vi "Proto Parser.vi"(8 "error in (no error)":errorcluster, 10 "Import Paths":path[](array[path]), 11 ".proto file path":path) -> (0 "error out":errorcluster, 1 "gRPC Method Parameters":T5[](array[typedef]), 2 "gRPC Enum Parameters":T1[](array[typedef]), 3 "gRPC Message Parameters":T2[](array[typedef]), 4 "Serialised Proto":string)   [LabVIEW 2019, in "gRPC Template Creation Utility.lvlib"]
uses:
  gRPC Template Creation Utility.lvlib
  TypeDefs/RPC Method Parameters.ctl
  TypeDefs/Message Metadata (Scripting).ctl
  TypeDefs/Message Element Metadata (Scripting).ctl
  TypeDefs/Message Element Type.ctl
  TypeDefs/Enum Metadata (Scripting).ctl
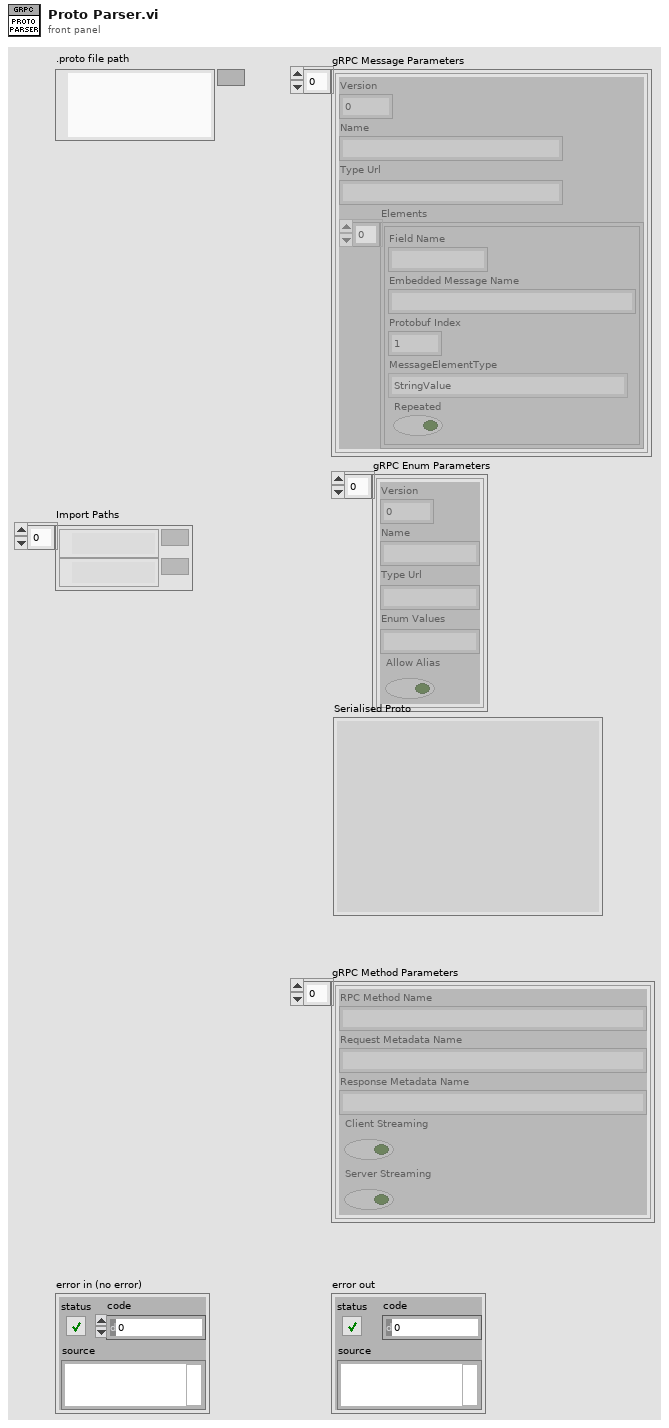
[diagram p1: front panel]
types:
  T1 = typedef "gRPC Template Creation Utility.lvlib/Enum Metadata (Scripting).ctl" = cluster{"Version":i32, "Name":string, "Type Url":string, "Enum Values":string, "Allow Alias":bool}
  T2 = typedef "gRPC Template Creation Utility.lvlib/Message Metadata (Scripting).ctl" = cluster{"Version":i32, "Name":string, "Type Url":string, "Elements":T3[]}
  T3 = typedef "gRPC Template Creation Utility.lvlib/Message Element Metadata (Scripting).ctl" = cluster{"Field Name":string, "Embedded Message Name":string, "Protobuf Index":i32, "MessageElementType":T4, "Repeated":bool}
  T4 = typedef "gRPC Template Creation Utility.lvlib/Message Element Type.ctl" = enum32{"Int32Value", "FloatValue", "DoubleValue", "BoolValue", "StringValue", "MessageValue", "Int64Value", "UInt32Value", "UInt64Value", "EnumValue", "Bytes", "Fixed64", "Fixed32", "SFixed64", "SFixed32", "SInt64", "SInt32"}
  T5 = typedef "gRPC Template Creation Utility.lvlib/RPC Method Parameters.ctl" = cluster{"RPC Method Name":string, "Request Metadata Name":string, "Response Metadata Name":string, "Client Streaming":bool, "Server Streaming":bool}
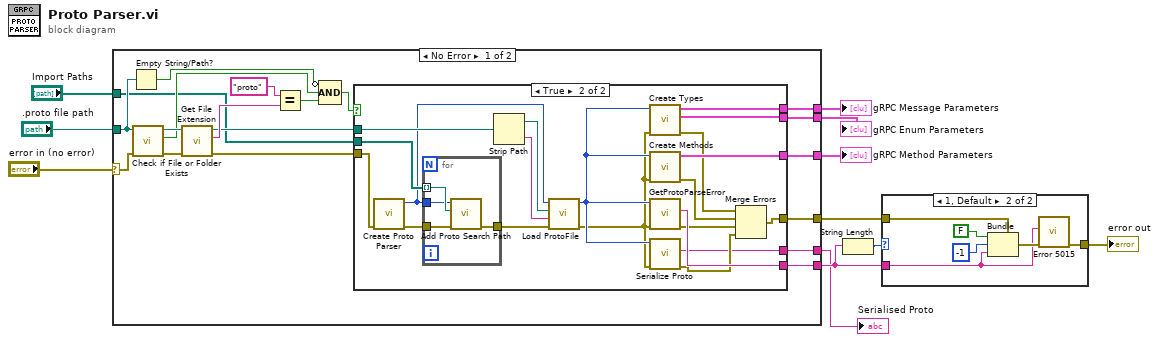
[diagram p0: block diagram]
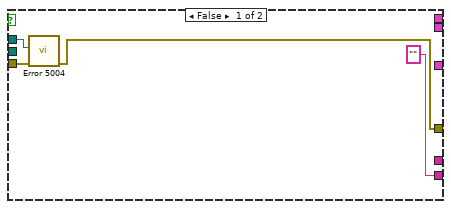
[diagram p3: hidden frame]
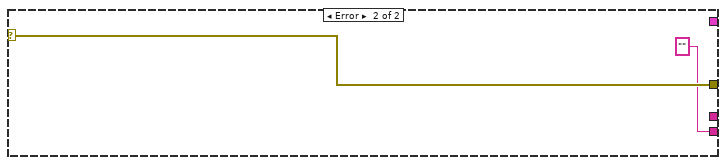
[diagram p4: hidden frame]
diagram:
  n1 = case shown="No Error" "error in (no error)" {
    selector: "error in (no error)" -> [w27 w60]
    tunnel: ".proto file path" -> [w28 _]
    tunnel: [w30 _] -> w11
    tunnel: [w29 w60] -> w5
    tunnel: [w16 _] -> w8
    tunnel: "Import Paths" -> [w15 _]
    tunnel: [w14 "" ("Error Message")] -> w3
    tunnel: [w13 _] -> w2
    tunnel: [w12 _] -> w1
    frame No Error {
      n2 = Empty String/Path?(string/path=w28) -> (empty?=w20:bool)
      n3 = call <vilib>:"Check if File or Folder Exists.vi"("error in (no error)"=w27, "path"=w28) -> ("error out"=w26:errorcluster, "file or folder exists?"=w21:bool, "dup path"=w25:path)  [unwired: 7 in]
      n4 = call <vilib>:"Get File Extension.vi"("error in (no error)"=w26, "file"=w25) -> ("error out"=w17:errorcluster, "lowercase file extension"=w24:string, "dup file"=w18:path)  [unwired: 5 in, 2 out]
      n5 = Equal?(x="proto", y=w24) -> (x = y?=w22:bool)
      n6 = Compound Arithmetic op=AND(invert w20, w21, w22) -> (w19:bool)
      n7 = case shown="True" w19 {
        tunnel: [_ w54] -> w30
        tunnel: [w33 w51] -> w29
        tunnel: w18 -> [w32 w53]
        tunnel: w17 -> [w34 w49]
        tunnel: [_ w42] -> w16
        tunnel: w15 -> [_ w48]
        tunnel: ["" ("Error Message") w44] -> w14
        tunnel: [_ w41] -> w13
        tunnel: [_ w35] -> w12
        frame False {
          n8 = call "Error 5004.vi"("error in (no error)"=w34, "Proto file path"=w32) -> ("error out"=w33:errorcluster)  [unwired: 9 in]
        }
        frame True {
          n9 = call "Create Proto Parser.vi"("error in (no error)"=w49) -> ("error out"=w47:errorcluster, "protoFile ref out"=w43:u64)  [unwired: 9 in]
          n10 = for {
            tunnel: w48 -> [w58] mode=indexing
            tunnel: w43 -> [w55]
            tunnel: w47 -> [w57]
            tunnel: [w56] -> w46
            n11 = call "Add Proto Search Path.vi"("error in (no error)"=w57, "Search Path"=w58, "protoFile ref in"=w55) -> ("error out"=w56:errorcluster)  [unwired: 7 in, 1 out]
          }
          n12 = Strip Path(path=w53) -> (stripped path=w45:path, name=w50:string)
          n13 = call "Load ProtoFile.vi"("protoFile ref in"=w43, "File Base path"=w45, "File Name"=w50, "error in (no error)"=w46) -> ("protoFile ref out"=w38:u64, "error out"=w37:errorcluster)  [unwired: 5 in]
          n14 = call "Create Types.vi"("error in (no error)"=w37, "protoFile ref in"=w38) -> ("error out"=w40:errorcluster, "Enum Parameters"=w41:T1[], "Message Parameters"=w42:T2[])  [unwired: 7 in]
          n15 = call "Create Methods.vi"("error in (no error)"=w37, "protoFile ref in"=w38) -> ("error out"=w52:errorcluster, "Method Parameters"=w54:T5[])  [unwired: 8 in]
          n16 = call "GetProtoParseError.vi"("error in (no error)"=w37, "Protofile ref in"=w38) -> ("error out"=w39:errorcluster, "Error Message"=w44:string)  [unwired: 7 in, 1 out]
          n17 = call "Serialize Proto.vi"("protoFile ref in"=w38, "error in (no error)"=w37) -> ("outBuffer"=w35:string, "error out"=w36:errorcluster)  [unwired: 6 in, 1 out]
          n18 = Merge Errors(w40, w52, w39, w36) -> (w51:errorcluster)
        }
      }
    }
    frame Error {
    }
  }
  "gRPC Method Parameters" <- w11
  "gRPC Message Parameters" <- w8
  "gRPC Enum Parameters" <- w2
  "Serialised Proto" <- w1
  n19 = String Length(string=w3) -> (length=w6:i32)
  n20 = case shown="1, Default" w6 {
    tunnel: w5 -> [w61 w67]
    tunnel: [w61 w62] -> w4
    tunnel: w3 -> [_ w63]
    frame 0 {
    }
    frame 1, Default {
      n21 = Bundle(cluster=w67, "status"=FALSE, "code"=-1, "source"=w63) -> (w64:errorcluster)
      n22 = call "Error 5015.vi"("error in (no error)"=w64, "Additional Error text"=w63) -> ("error out"=w62:errorcluster)  [unwired: 9 in]
    }
  }
  "error out" <- w4
